vi "Get_BodyDim.vi"(8 "error in (no error)":errorcluster, 11 "CAlexData in":refnum<class "CAlex2_Data.lvclass">) -> (0 "error out":errorcluster, 2 "BodyDim(m)":T1, 3 "CAlexData out":refnum<class "CAlex2_Data.lvclass">)   [LabVIEW 2016, in "CAlex2_Data.lvclass"]
uses:
  CAlex2_Data.lvclass
  CAlex2_Data.lvclass/CAlex2_Data.ctl
  Classes/CAlex2/CAlex2.lvclass
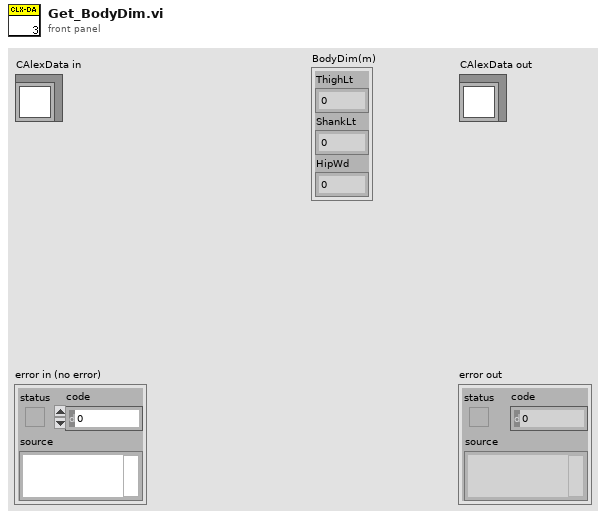
[diagram p1: front panel]
types:
  T1 = cluster{"ThighLt":dbl, "ShankLt":dbl, "HipWd":dbl}
  T2 = typedef "CAlex2.lvclass/LowerBodyDim.ctl" = cluster{"BodyDim":cluster{"ThighLt (m)":dbl, "ShankLt (m)":dbl, "HipWd (m)":dbl}, "BodyWt":cluster{"Thigh (kg)":dbl, "Shank (kg)":dbl}, "Cuff Loc":cluster{"HipCuffWd (m)":dbl, "HipCuffHt (m)":dbl, "HipFwdShift (m)":dbl, "ThighToKnee (m)":dbl, "ThighCuffDist (m)":dbl, "ShankToKnee (m)":dbl}}
  T3 = cluster{"ThighLt (m)":dbl, "ShankLt (m)":dbl, "HipWd (m)":dbl}
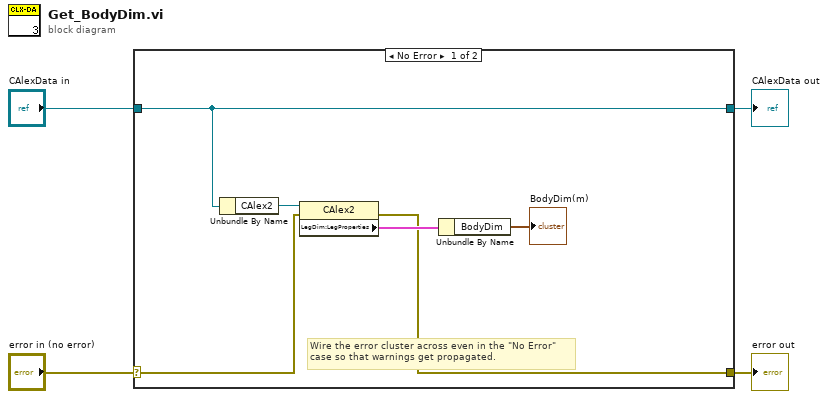
[diagram p0: block diagram]
diagram:
  n1 = case shown="No Error" "error in (no error)" {
    selector: "error in (no error)" -> [w7 w12]
    tunnel: [w6 w12] -> w3
    tunnel: [w10 w11] -> w1
    tunnel: "CAlexData in" -> [w10 w11]
    frame No Error {
      # "Wire the error cluster across even in the \"No Error\"\ncase so that warnings get propagated."
      n2 = Unbundle By Name(w10) -> ("CAlex2"=w9:refnum<class "CAlex2.lvclass">)
      n3 = property class="CAlex2"(reference=w9, error in=w7) -> (error out=w6:errorcluster, "LegDim:LegProperties"=w8:T2)  [unwired: 1 out]
      n4 = Unbundle By Name(w8) -> ("BodyDim"=→"BodyDim(m)":T3)
    }
    frame Error {
    }
  }
  "error out" <- w3
  "CAlexData out" <- w1
